vi "Pre Launch Init.vi"(11 "SCADA Communications in":refnum<class "SCADA Communications.lvclass">) -> (0 "error out":errorcluster, 3 "SCADA Communications out":refnum<class "SCADA Communications.lvclass">)   [LabVIEW 2015, in "SCADA Communcations Actor.lvlib" / "SCADA Communications.lvclass"]
doc: "(<B>Filename</B>: Actor Framework.lvlib:Actor.lvclass:Pre Launch Init.vi)\n\nDefines behavior that occurs after the Launch Nested Actor method is invoked but before the actor's Actor Core method begins running.\n\nBy default, this method does nothing. A descendant class may override it to define behavior."
uses:
  SCADA Communications.lvclass
  SCADA Communications Messages/Read Packet Msg/Read Packet Msg.lvclass
  SCADA Communications.lvclass/SCADA Communications.ctl
  TCPIP Communications Framework/TCPIP Communications/TCPIP Communications.lvclass
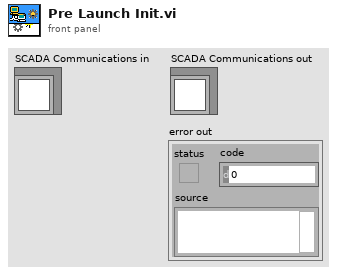
[diagram p1: front panel]
types:
  T1 = typedef "SCADA Communcations Actor.lvlib/SCADA Communications.lvclass/Notifiers Cluster.ctl" = cluster{"stop":refnum<notifier>, "Comms stop":refnum<notifier>}
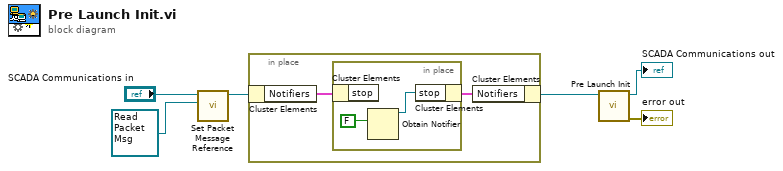
[diagram p0: block diagram]
diagram:
  n1 = call "Set Packet Message Reference.vi"("Packet Msg"=refnum<class "Read Packet Msg.lvclass"> refnum ("SCADA Communcations Actor.lvlib:Read Packet Msg.lvclass"), "TCPIP Communications in"="SCADA Communications in") -> ("TCPIP Communications out"=w3:refnum<class "SCADA Communications.lvclass">)  [unwired: 9 in]
  n2 = in-place {
    n3 = in-place-cluster #1(w3) -> ("Notifiers"=w8:T1)
    n4 = in-place {
      n5 = in-place-cluster #2(w8) -> ()  [unwired: 1 out]
      n6 = Obtain Notifier(notification data type=FALSE) -> (notifier out=w9:refnum<notifier>)  [unwired: 3 in, 2 out]
      n7 = in-place-cluster #2("stop"=w9) -> (w7:T1)
    }
    n8 = in-place-cluster #1("Notifiers"=w7) -> (w2:refnum<class "SCADA Communications.lvclass">)
  }
  n9 = call-parent "Pre Launch Init.vi"("TCPIP Communications in"=w2) -> ("error out"=→"error out":errorcluster, "TCPIP Communications out"=→"SCADA Communications out":refnum<class "SCADA Communications.lvclass">)  [unwired: 9 in]
